vi "read_counter_old.vi"() -> ()   [LabVIEW 2011]
panel:
  out "data out":string
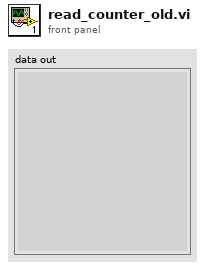
[diagram p1: front panel]
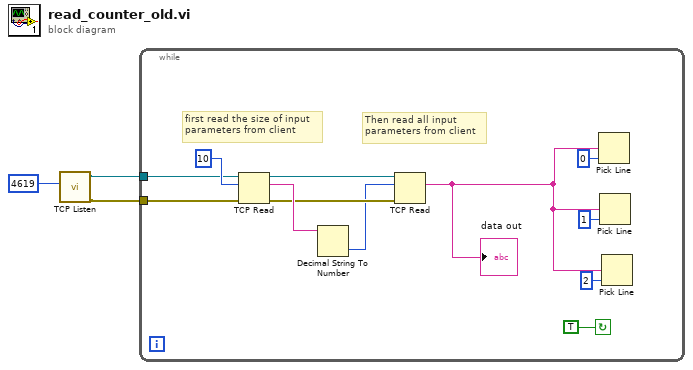
[diagram p0: block diagram]
diagram:
  n1 = call <vilib>:"TCP Listen.vi"("port"=u16 4619) -> ("error out"=w1:errorcluster, "connection ID"=w2:refnum<k5>)  [unwired: 6 in, 3 out]
  n2 = while {
    tunnel: w2 -> [w9]
    tunnel: w1 -> [w8]
    stop <- TRUE continue-if-true
    # "Then read all input \nparameters from client"
    # "first read the size of input \nparameters from client"
    n3 = TCP Read(connection ID=w9, bytes to read=10, error in (no error)=w8) -> (connection ID out=w12:refnum<k5>, data out=w13:string, error out=w11:errorcluster)  [unwired: 2 in]
    n4 = Decimal String To Number(string=w13) -> (number=w10:i32)  [unwired: 2 in, 1 out]
    n5 = TCP Read(connection ID=w12, bytes to read=w10, error in (no error)=w11) -> (data out=w6:string)  [unwired: 2 in, 2 out]
    "data out" <- w6
    n6 = Pick Line(multi-line string=w6, line index=0) -> ()  [unwired: 1 in, 1 out]
    n7 = Pick Line(multi-line string=w6, line index=1) -> ()  [unwired: 1 in, 1 out]
    n8 = Pick Line(multi-line string=w6, line index=2) -> ()  [unwired: 1 in, 1 out]
  }
